vi "Test Minimal Audio Device Capture.vi"(8 "error in (no error)":errorcluster) -> (0 "error out":errorcluster, 3 "Pass?":bool)   [LabVIEW 2020]
uses:
  G-Audio/Controls/Audio Device Info.ctl
  G-Audio/Controls/Audio Device Type.ctl
  8ac02ed0-e0ad-414e-8015-75faf73f9d75.vi
  G-Audio/Private/Result To Error.vi
  8ac02ed0-e0ad-414e-8015-75faf73f9d75.vi/6b901882-6109-4f44-aca5-48e1525e5248.vi
  8ac02ed0-e0ad-414e-8015-75faf73f9d75.vi/06c0137a-63d3-4e30-982f-115d83a1188c.vi
  G-Audio/Private/Get Configured Audio Device Info.vi
  8ac02ed0-e0ad-414e-8015-75faf73f9d75.vi/06c0137a-63d3-4e30-982f-115d83a1188c.vi/4b7b629c-2e91-4160-9820-a26af8f6e677.vi
  <vilib>/Utility/Data Type/Get Numeric Information.vi
  <vilib>/Utility/error.llb/Error Cluster From Error Code.vi
  G-Audio/G-Audio.lvlib
panel:
  out "Waveform Graph":waveform(i16)[](graph)
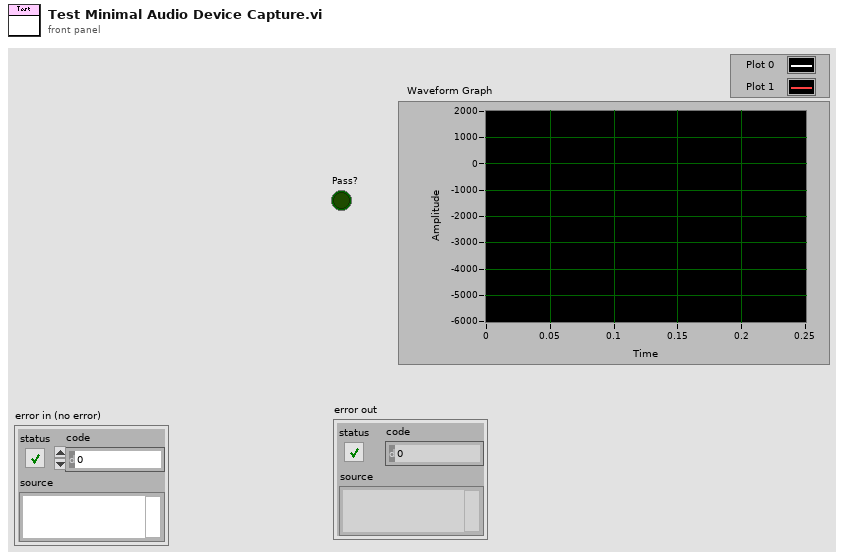
[diagram p1: front panel]
types:
  T1 = typedef "G-Audio.lvlib/Audio Device Info.ctl" = cluster{"Name":string, "ID":u8[], "Device Type":T2}
  T2 = typedef "G-Audio.lvlib/Audio Device Type.ctl" = enum16{"(None)", "Playback", "Capture", "Duplex", "Loopback"}
  T3 = typedef "G-Audio.lvlib/Audio Device Refnum.ctl" = refnum<file>
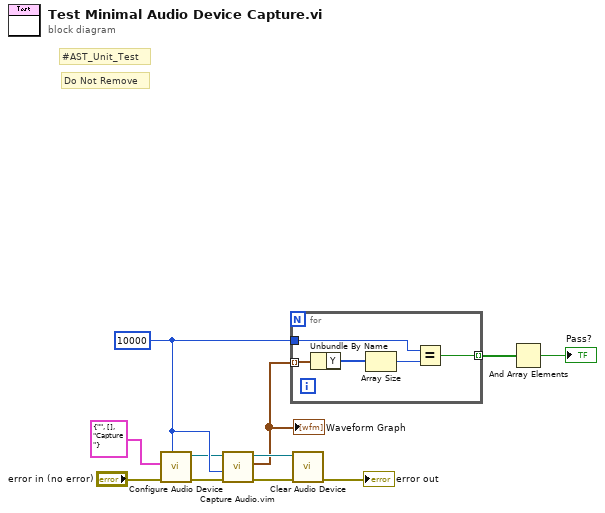
[diagram p0: block diagram]
diagram:
  w11 = 10000
  # "Do Not Remove"
  # "#AST_Unit_Test"
  n1 = call "Configure Audio Device.vi"("Buffer Size (4096)"=w11, "error in (no error)"="error in (no error)", "Audio Device"=T1 {"Name"="", "ID"=[], "Device Type"=enum."Capture"}) -> ("error out"=w7:errorcluster, "Audio Device Refnum"=w8:T3)  [unwired: 7 in]
  n2 = call "Capture Audio.vim"("error in (no error)"=w7, "Samples To Read"=w11, "Audio Device Refnum In"=w8) -> ("error out"=w4:errorcluster, "Audio Data"=w3:waveform(i16)[], "Audio Device Refnum Out"=w5:T3)  [unwired: 6 in]
  "Waveform Graph" <- w3
  n3 = for {
    tunnel: w3 -> [w16] mode=indexing
    tunnel: w11 -> [w14]
    tunnel: [w12] -> w10 mode=indexing
    n4 = Unbundle By Name(w16) -> ("Y"=w15:i16[])
    n5 = Array Size(array=w15) -> (size(s)=w13:i32)
    n6 = Equal?(x=w14, y=w13) -> (x = y?=w12:bool)
  }
  n7 = call "Clear Audio Device.vi"("error in (no error)"=w4, "Audio Device Refnum In"=w5) -> ("error out"=→"error out":errorcluster)  [unwired: 9 in]
  n8 = And Array Elements(Boolean array=w10) -> (logical AND=→"Pass?":bool)
